vi "Main RLC.vi"() -> ()   [LabVIEW 2017]
uses:
  Types/Parameters Values Type.ctl
  Data Share Type.ctl
  <vilib>/picture/picture.llb/imagedata.ctl
  Types/Parameters Names Type.ctl
  Types/Circuit Type Enum.ctl
  Types/Attachments Type.ctl
  Types/Id Type.ctl
panel:
  out "PUT Response body":string
  out "PUT Responce headers":string
  out "API PUT Endpoint Url Real":string
  out "PUT JSON Payload":string
  in  "API PUT Endpoint Url Pattern":string="https://api.dev.enlil.io/api/v1/document_revisions/external/document-revision-id"
  out "Serial file POST Responce headers":string
  out "Parallel file POST Responce headers":string
  in  "API POST Endpoint Url":string="https://api.dev.enlil.io/api/v1/attachments/external/upload"
  in  "Post Button":bool
  in  "Serial circuit fIlepath":path=path "E:/upwork/Labview-REST-API/serial.png"
  in  "Parallel circuit fIlepath":path=path "E:/upwork/Labview-REST-API/parallel.png"
  in  "Save Button":bool
  out "Serial - Frequency Response Picture":picture
  out "Parallel - Frequency Response Picture":picture
  in  "Calculate Button":bool
  out "Parameters Values":T1
  in  "API Token":string="apitoken 2096a662-4947-42f5-97bc-84cfdf20fe4e:bc240510-8f48-43e3-889a-471659905c2e"
  in  "API GET Endpoint Url":string="https://api.dev.enlil.io/api/v1/document_revisions/external/ALI00017/draft"
  in  "Get Button":bool
  in  "Close Button":bool
  # "1. GET request to receive filter parameters"
  # "2. Calculate Parallel/Serial circuits frequency responce"
  # "3. Save to file"
  # "4. POST/PUT requests to send images"
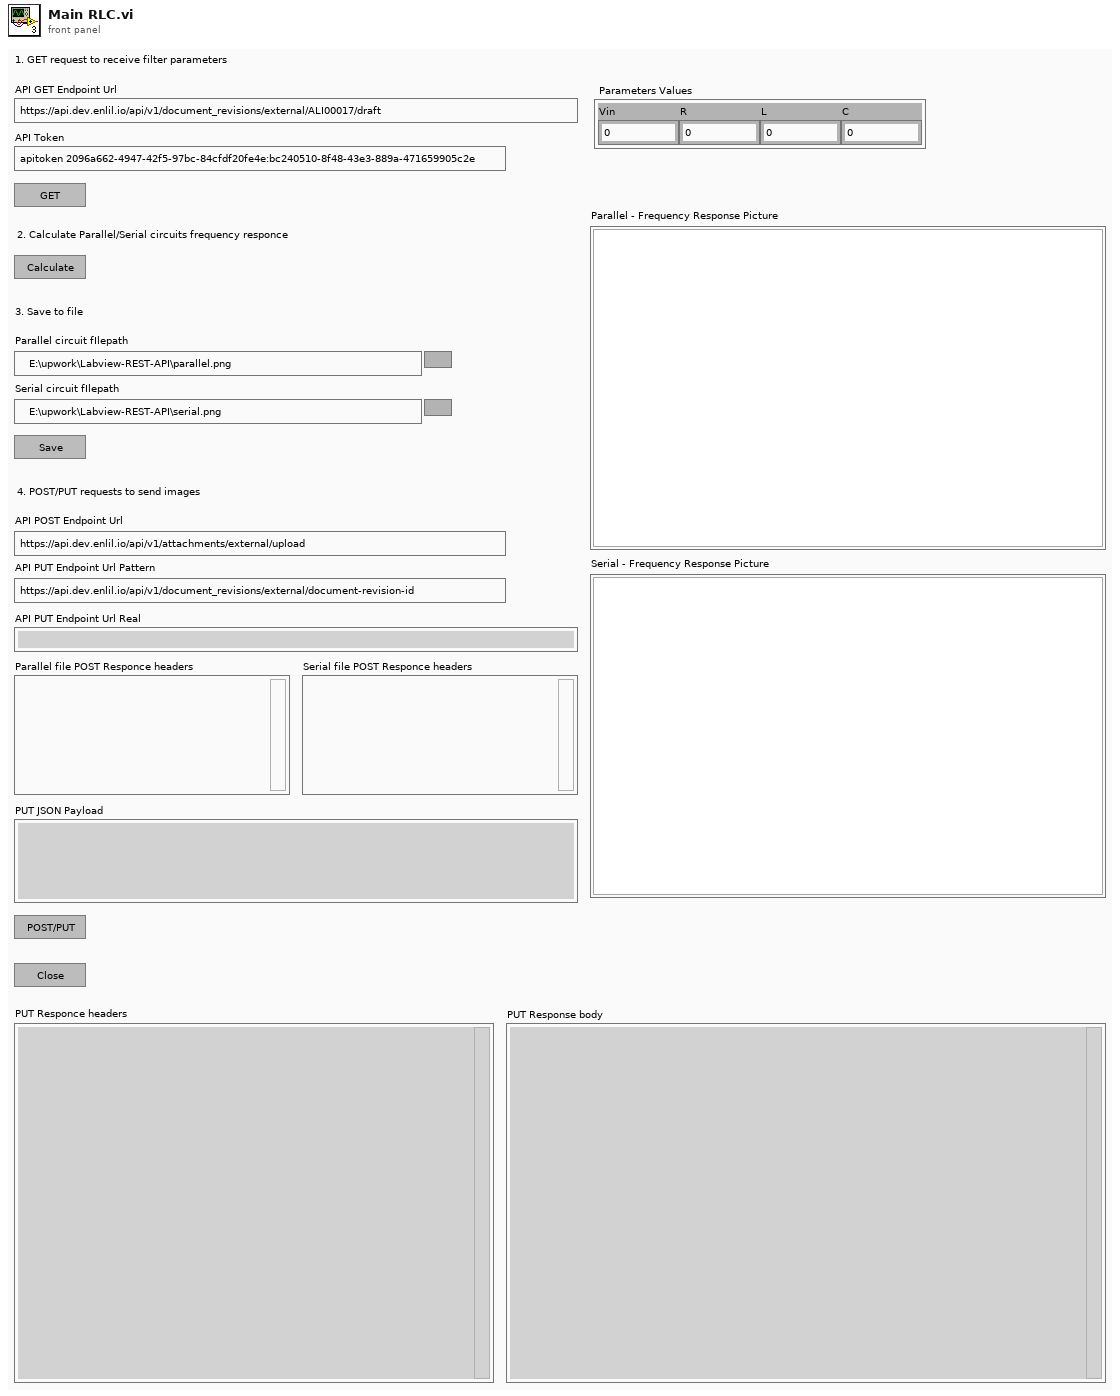
[diagram p1: front panel]
types:
  T1 = typedef "Parameters Values Type.ctl" = cluster{"Vin":dbl, "R":dbl, "L":dbl, "C":dbl}
  T2 = typedef "Data Share Type.ctl" = cluster{"Parallel Image Data":T3, "Serial Image Data":T3, "Parameters Values":T1, "Parallel circuit fIlepath":path, "Serial circuit fIlepath":path, "Document Id":string, "Parallel File Id":string, "Serial File Id":string, "Api Token":string}
  T3 = typedef "imagedata.ctl" = cluster{"image type":i32, "image depth":i32, "image":u8[], "mask":u8[], "colors":u32[], "Rectangle":cluster{"left":i16, "top":i16, "right":i16, "bottom":i16}}
  T4 = typedef "Parameters Names Type.ctl" = cluster{"Vin":string, "R":string, "L":string, "C":string}
  T5 = typedef "Circuit Type Enum.ctl" = enum16{"Parallel", "Serial"}
  T6 = typedef "Id Type.ctl" = cluster{"id":string}
  T7 = typedef "Attachments Type.ctl" = cluster{"attachments":T6[]}
  T8 = typedef "Body Parameter Type.ctl" = cluster{"Name":string, "Value":string}
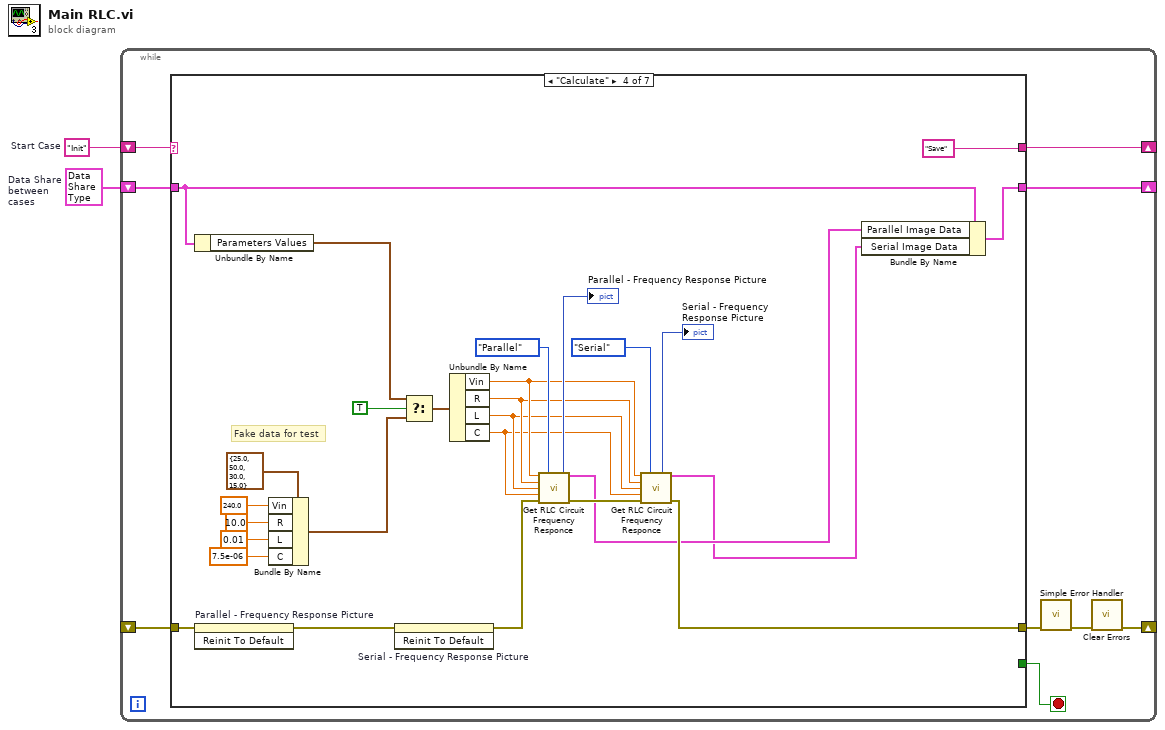
[diagram p0: block diagram]
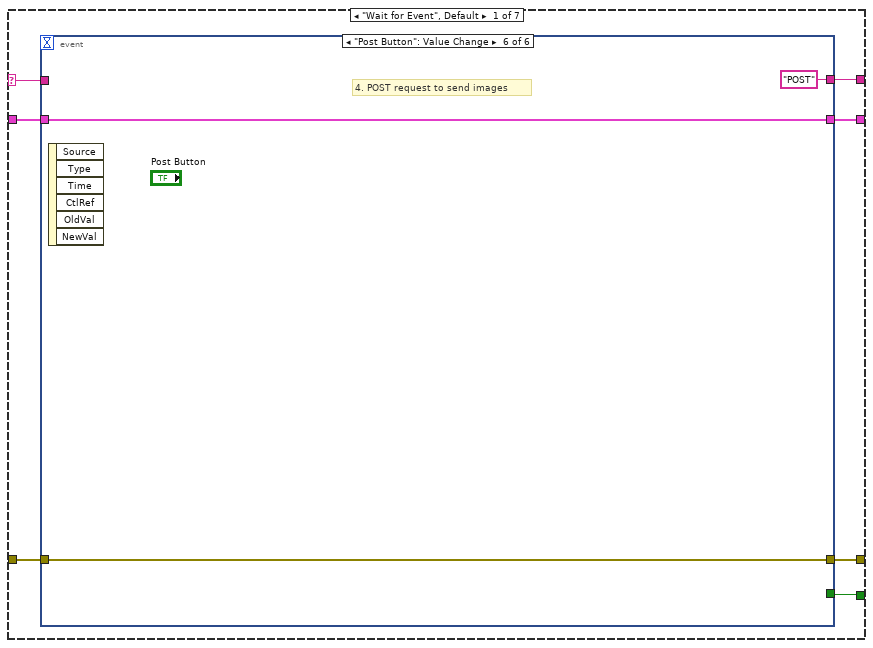
[diagram p2: hidden frame]
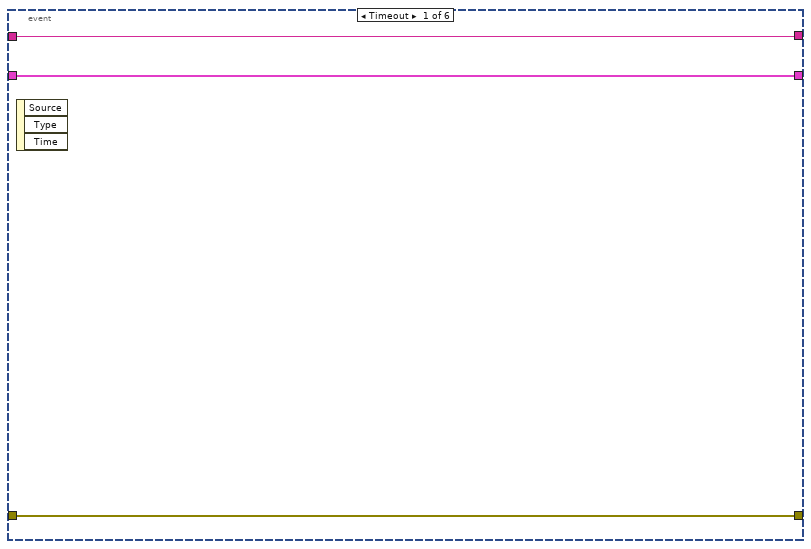
[diagram p3: hidden frame]
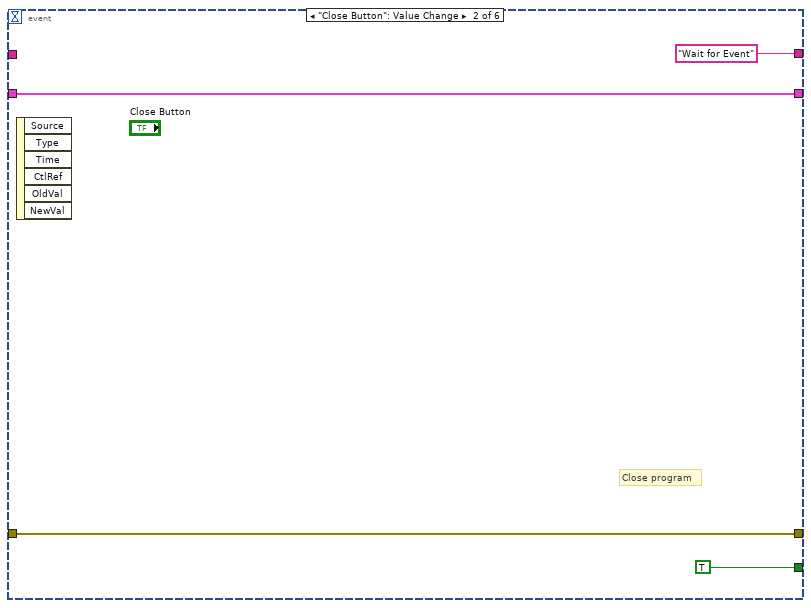
[diagram p4: hidden frame]
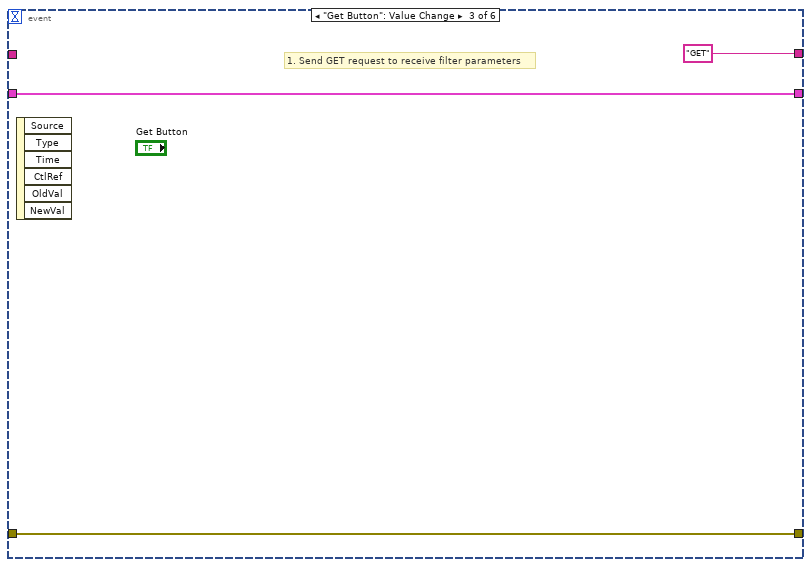
[diagram p5: hidden frame]
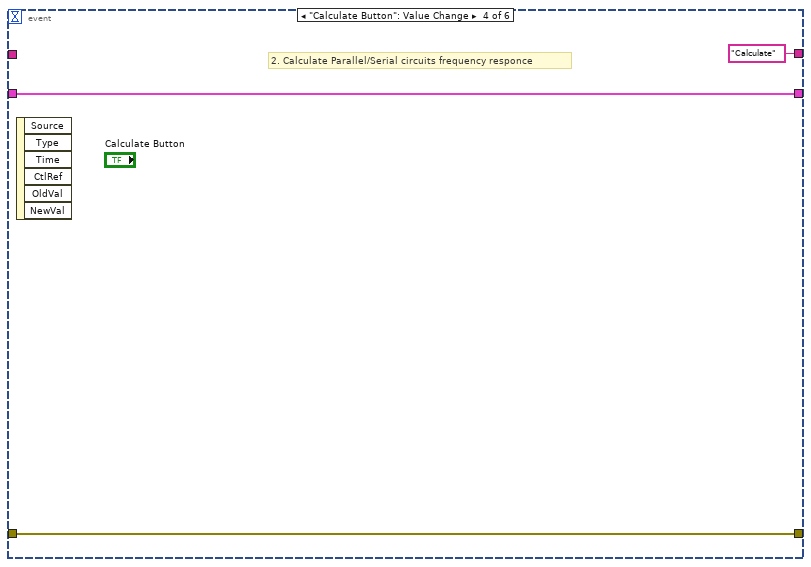
[diagram p6: hidden frame]
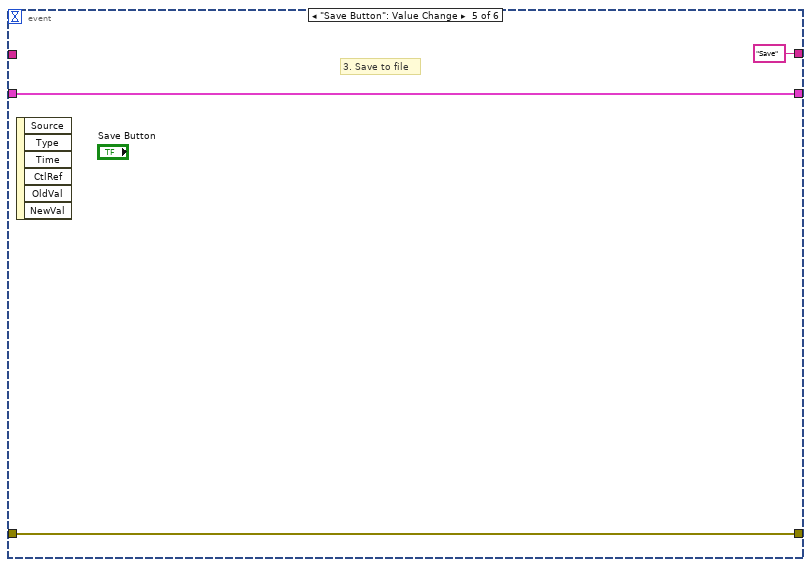
[diagram p7: hidden frame]
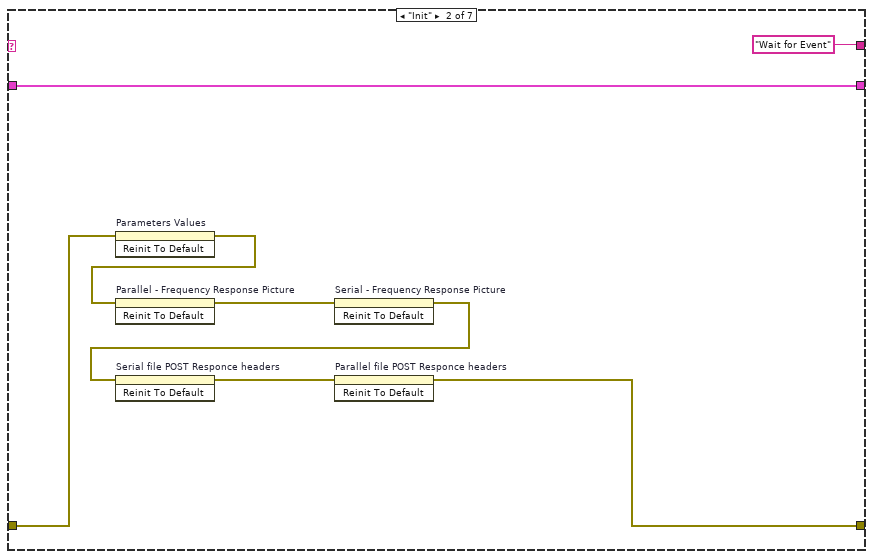
[diagram p8: hidden frame]
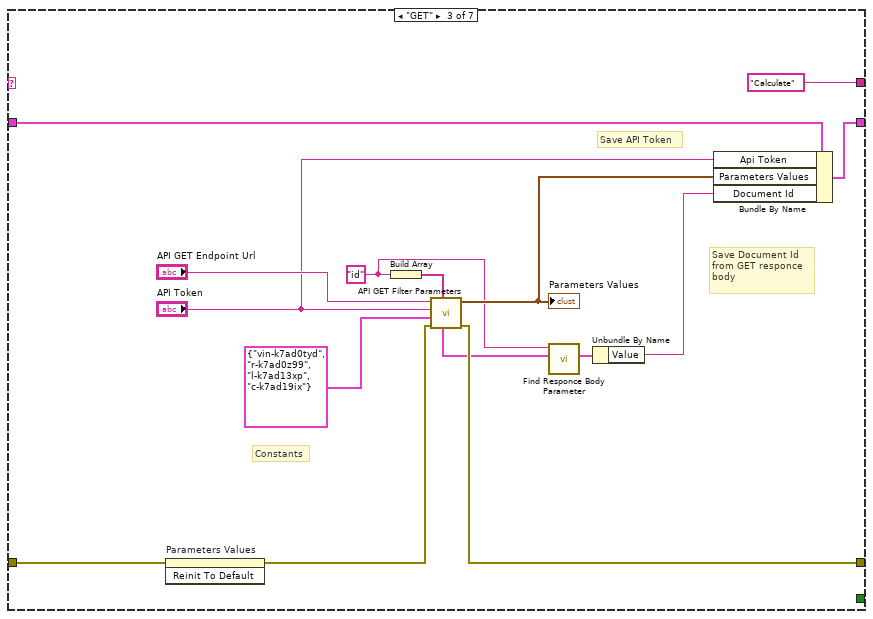
[diagram p9: hidden frame]
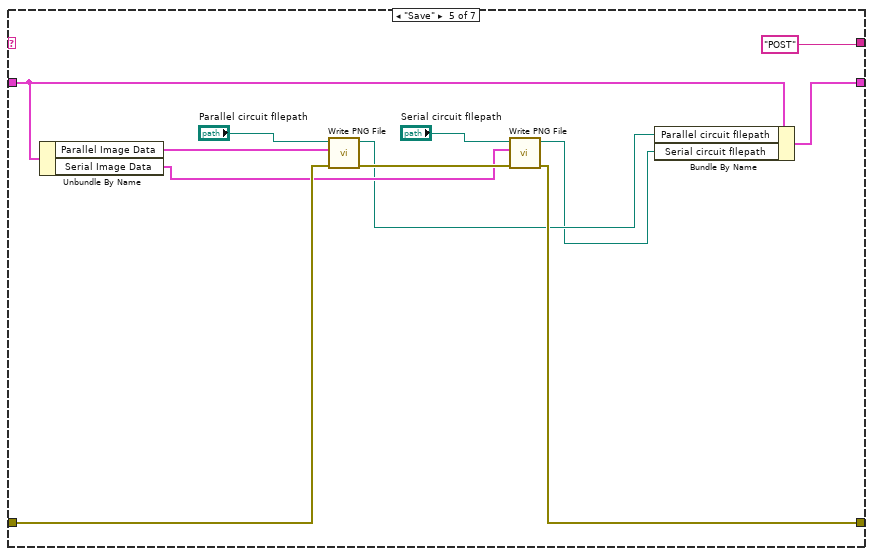
[diagram p10: hidden frame]
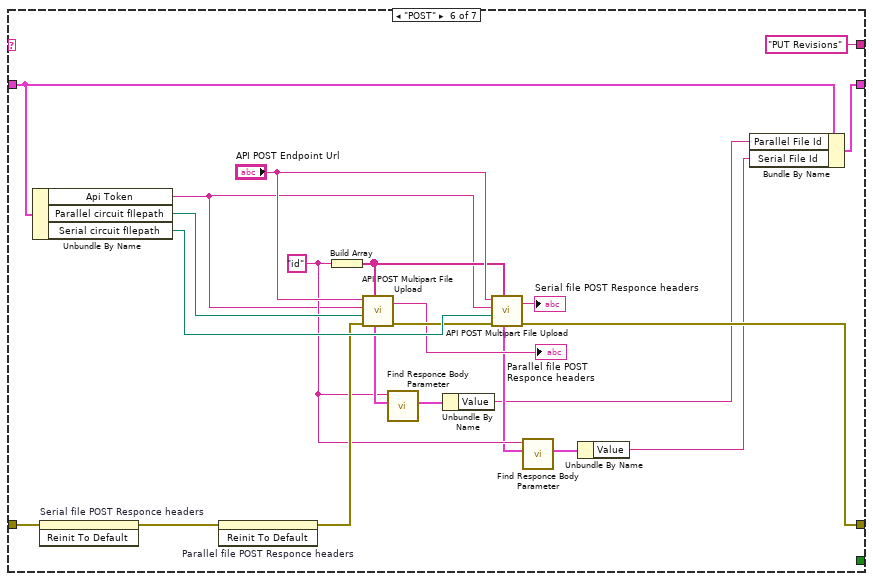
[diagram p11: hidden frame]
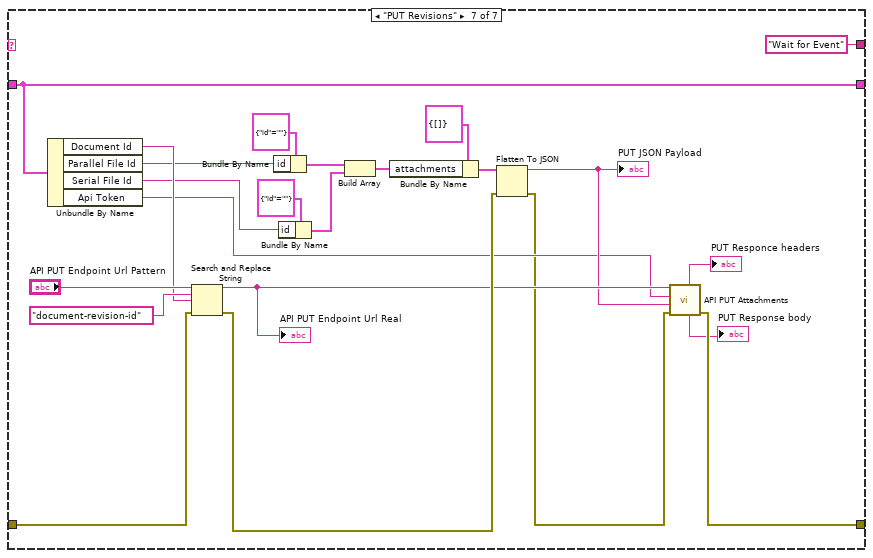
[diagram p12: hidden frame]
diagram:
  w1 = T2 {"Parallel Image Data"={"image type"=0, "image depth"=0, "image"=[], "mask"=[], "colors"=[], "Rectangle"={"left"=0, "top"=0, "right"=0, "bottom"=0}}, "Serial Image Data"={"image type"=0, "image depth"=0, "image"=[], "mask"=[], "colors"=[], "Rectangle"={"left"=0, "top"=0, "right"=0, "bottom"=0}}, "Parameters Values"={"Vin"=0.0, "R"=0.0, "L"=0.0, "C"=0.0}, "Parallel circuit fIlepath"=path "D:/upwork/Labview-REST-API/parallel.png", "Serial circuit fIlepath"=path "D:/upwork/Labview-REST-API/serial.png", "Document Id"="", "Parallel File Id"="", "Serial File Id"="", "Api Token"=""}  # Data Share between  cases
  w2 = "Init"  # Start Case
  n1 = while {
    shift-right: [w9] -> _
    shift-left: w2 -> [w11]
    shift-right: [w5] -> _
    shift-left: _ -> [w8]
    shift-right: [w3] -> _
    shift-left: w1 -> [w4]
    stop <- w10 stop-if-true
    n2 = case shown="\"Calculate\"" w11 {
      selector: w11 -> [w17 _ _ _ _ _ _]
      tunnel: [w18 _ _ _ _ _ _] -> w10
      tunnel: [w16 "Wait for Event" "Calculate" "Save" "POST" "PUT Revisions" "Wait for Event"] -> w9
      tunnel: [w14 w38 w57 w83 w92 w116 w124] -> w7
      tunnel: w8 -> [w15 w44 w56 w82 w96 w113 w130]
      tunnel: w4 -> [w13 w42 w54 w64 w90 w104 w141]
      tunnel: [w12 w42 w53 w63 w91 w103 w141] -> w3
      frame "Wait for Event", Default {
        n3 = event shown="[5] \"Post Button\": Value Change" {
          selector: _ -> [_ _ _ _ _ _]
          dyn-events: _ -> [_ _ _ _ _ _]
          timeout: _ -> [_ _ _ _ _ _]
          tunnel: [_ TRUE _ _ _ _] -> w18
          tunnel: w17 -> [w21 _ _ _ _ _]
          tunnel: [w21 "Wait for Event" "GET" "Calculate" "Save" "POST"] -> w16
          tunnel: w15 -> [w20 w23 w27 w30 w32 w35]
          tunnel: [w20 w23 w27 w30 w32 w35] -> w14
          tunnel: w13 -> [w19 w22 w26 w29 w33 w36]
          tunnel: [w19 w22 w26 w29 w33 w36] -> w12
          event Timeout {
            n4 = event-data() -> ()  [unwired: 1 in, 3 out]
          }
          event "Close Button": Value Change {
            # "Close program"
            n5 = event-data() -> ()  [unwired: 1 in, 6 out]
          }
          event "Get Button": Value Change {
            # "1. Send GET request to receive filter parameters"
            n6 = event-data() -> ()  [unwired: 1 in, 6 out]
          }
          event "Calculate Button": Value Change {
            # "2. Calculate Parallel/Serial circuits frequency responce"
            n7 = event-data() -> ()  [unwired: 1 in, 6 out]
          }
          event "Save Button": Value Change {
            # "3. Save to file"
            n8 = event-data() -> ()  [unwired: 1 in, 6 out]
          }
          event "Post Button": Value Change {
            # "4. POST request to send images"
            n9 = event-data() -> ()  [unwired: 1 in, 6 out]
          }
        }
      }
      frame "Init" {
        n10 = invoke on="Parameters Values" class="Clust (strict)" method="Reinit To Default"(error in=w44) -> (error out=w41:errorcluster)  [unwired: 2 in, 2 out]
        n11 = invoke on="Parallel - Frequency Response Picture" class="Pict" method="Reinit To Default"(error in=w41) -> (error out=w43:errorcluster)  [unwired: 2 in, 2 out]
        n12 = invoke on="Serial - Frequency Response Picture" class="Pict" method="Reinit To Default"(error in=w43) -> (error out=w39:errorcluster)  [unwired: 2 in, 2 out]
        n13 = invoke on="Serial file POST Responce headers" class="Str" method="Reinit To Default"(error in=w39) -> (error out=w40:errorcluster)  [unwired: 2 in, 2 out]
        n14 = invoke on="Parallel file POST Responce headers" class="Str" method="Reinit To Default"(error in=w40) -> (error out=w38:errorcluster)  [unwired: 2 in, 2 out]
      }
      frame "GET" {
        w49 = "id" ("String")
        # "Save Document Id\nfrom GET responce\nbody"
        # "Save API Token"
        # "Constants"
        n15 = invoke on="Parameters Values" class="Clust (strict)" method="Reinit To Default"(error in=w56) -> (error out=w55:errorcluster)  [unwired: 2 in, 2 out]
        n16 = Build Array(w49) -> (w50:string[])
        n17 = call "API GET Filter Parameters.vi"("Body Parameters Names"=w50, "error in (no error)"=w55, "Filter Parameters Names"=T4 {"Vin"="vin-k7ad0tyd", "R"="r-k7ad0z99", "L"="l-k7ad13xp", "C"="c-k7ad19ix"} ("Parameters Names"), "API Token"="API Token", "API Endpoint Url"="API GET Endpoint Url") -> ("error out"=w57:errorcluster, "Parameters Values"=w52:T1, "Body Parameters out"=w51:T8[])  [unwired: 2 in, 2 out]
        "Parameters Values" <- w52
        n18 = call "Find Responce Body Parameter.vi"("Body Parameters in"=w51, "Parameter name"=w49) -> ("Body Parameter"=w48:T8)  [unwired: 8 in, 1 out]
        n19 = Unbundle By Name(w48) -> ("Value"=w47:string)
        n20 = Bundle By Name(cluster=w54, "Api Token"="API Token", "Parameters Values"=w52, "Document Id"=w47) -> (w53:T2)
      }
      frame "Calculate" {
        # "Fake data for test"
        n21 = Unbundle By Name(w64) -> ("Parameters Values"=w65:T1)
        n22 = invoke on="Parallel - Frequency Response Picture" class="Pict" method="Reinit To Default"(error in=w82) -> (error out=w81:errorcluster)  [unwired: 2 in, 2 out]
        n23 = Bundle By Name(cluster=T1 {"Vin"=25.0, "R"=50.0, "L"=30.0, "C"=15.0} ("Parameters Values"), "Vin"=240.0, "R"=10.0, "L"=0.01, "C"=7.5e-06) -> (w68:T1)
        n24 = invoke on="Serial - Frequency Response Picture" class="Pict" method="Reinit To Default"(error in=w81) -> (error out=w80:errorcluster)  [unwired: 2 in, 2 out]
        n25 = Select(t=w65, s=TRUE, f=w68) -> (s? t:f=w67:T1)
        n26 = Unbundle By Name(w67) -> ("Vin"=w79:dbl, "R"=w78:dbl, "L"=w77:dbl, "C"=w76:dbl)
        n27 = call "Get RLC Circuit Frequency Responce.vi"("Vin amplitude"=w79, "Circuit Type Enum"=Circuit_Type_Enum."Parallel", "Resistence (R)"=w78, "Impedence (H)"=w77, "Capacitave (F)"=w76, "error in (no error)"=w80) -> ("Frequency Response Picture"=→"Parallel - Frequency Response Picture":picture, "Frequency Response Image Data"=w62:T3, "error out"=w84:errorcluster)  [unwired: 6 in, 1 out]
        n28 = call "Get RLC Circuit Frequency Responce.vi"("Vin amplitude"=w79, "Circuit Type Enum"=Circuit_Type_Enum."Serial", "Resistence (R)"=w78, "Impedence (H)"=w77, "Capacitave (F)"=w76, "error in (no error)"=w84) -> ("Frequency Response Picture"=→"Serial - Frequency Response Picture":picture, "Frequency Response Image Data"=w61:T3, "error out"=w83:errorcluster)  [unwired: 6 in, 1 out]
        n29 = Bundle By Name(cluster=w64, "Parallel Image Data"=w62, "Serial Image Data"=w61) -> (w63:T2)
      }
      frame "Save" {
        n30 = Unbundle By Name(w90) -> ("Parallel Image Data"=w97:T3, "Serial Image Data"=w93:T3)
        n31 = call <vilib>:"Write PNG File.vi"("error in (no error)"=w96, "image data"=w97, "path to PNG file"="Parallel circuit fIlepath") -> ("error out"=w95:errorcluster, "path"=w89:path)  [unwired: 7 in]
        n32 = call <vilib>:"Write PNG File.vi"("error in (no error)"=w95, "image data"=w93, "path to PNG file"="Serial circuit fIlepath") -> ("error out"=w92:errorcluster, "path"=w88:path)  [unwired: 7 in]
        n33 = Bundle By Name(cluster=w90, "Parallel circuit fIlepath"=w89, "Serial circuit fIlepath"=w88) -> (w91:T2)
      }
      frame "POST" {
        w106 = "id" ("String")
        n34 = Unbundle By Name(w104) -> ("Api Token"=w100:string, "Parallel circuit fIlepath"=w120:path, "Serial circuit fIlepath"=w118:path)
        n35 = invoke on="Serial file POST Responce headers" class="Str" method="Reinit To Default"(error in=w113) -> (error out=w112:errorcluster)  [unwired: 2 in, 2 out]
        n36 = invoke on="Parallel file POST Responce headers" class="Str" method="Reinit To Default"(error in=w112) -> (error out=w111:errorcluster)  [unwired: 2 in, 2 out]
        n37 = Build Array(w106) -> (w110:string[])
        n38 = call "API POST Multipart File Upload.vi"("Body Parameters Names"=w110, "error in (no error)"=w111, "FIlepath"=w120, "API Token"=w100, "API Endpoint Url"="API POST Endpoint Url") -> ("error out"=w117:errorcluster, "Responce headers"=→"Parallel file POST Responce headers":string, "Body Parameters out"=w109:T8[])  [unwired: 3 in, 1 out]
        n39 = call "Find Responce Body Parameter.vi"("Body Parameters in"=w109, "Parameter name"=w106) -> ("Body Parameter"=w108:T8)  [unwired: 8 in, 1 out]
        n40 = Unbundle By Name(w108) -> ("Value"=w102:string)
        n41 = call "API POST Multipart File Upload.vi"("Body Parameters Names"=w110, "error in (no error)"=w117, "FIlepath"=w118, "API Token"=w100, "API Endpoint Url"="API POST Endpoint Url") -> ("error out"=w116:errorcluster, "Responce headers"=→"Serial file POST Responce headers":string, "Body Parameters out"=w105:T8[])  [unwired: 3 in, 1 out]
        n42 = call "Find Responce Body Parameter.vi"("Body Parameters in"=w105, "Parameter name"=w106) -> ("Body Parameter"=w107:T8)  [unwired: 8 in, 1 out]
        n43 = Unbundle By Name(w107) -> ("Value"=w101:string)
        n44 = Bundle By Name(cluster=w104, "Parallel File Id"=w102, "Serial File Id"=w101) -> (w103:T2)
      }
      frame "PUT Revisions" {
        n45 = Unbundle By Name(w141) -> ("Document Id"=w140:string, "Parallel File Id"=w137:string, "Serial File Id"=w135:string, "Api Token"=w126:string)
        n46 = Search and Replace String(input string="API PUT Endpoint Url Pattern", search string="document-revision-id", replace string=w140, error in=w130) -> (result string=w128:string, error out=w129:errorcluster)  [unwired: 4 in, 2 out]
        "API PUT Endpoint Url Real" <- w128
        n47 = Bundle By Name(cluster=T6 {"id"=""} ("Id Type"), "id"=w137) -> (w134:T6)
        n48 = Bundle By Name(cluster=T6 {"id"=""} ("Id Type"), "id"=w135) -> (w133:T6)
        n49 = Build Array(w134, w133) -> (w132:T6[])
        n50 = Bundle By Name(cluster=T7 {"attachments"=[]} ("Attachments Type"), "attachments"=w132) -> (w131:T7)
        n51 = Flatten To JSON(anything=w131, error in (no error)=w129) -> (JSON string=w127:string, 11:w125:errorcluster)  [unwired: 1 in]
        "PUT JSON Payload" <- w127
        n52 = call "API PUT Attachments.vi"("error in (no error)"=w125, "Buffer"=w127, "API Token"=w126, "API Endpoint Url"=w128) -> ("error out"=w124:errorcluster, "Response body"=→"PUT Response body":string, "Responce headers"=→"PUT Responce headers":string)  [unwired: 5 in]
      }
    }
    n53 = call <vilib>:"Simple Error Handler.vi"("error in (no error)"=w7) -> ("error out"=w6:errorcluster)  [unwired: 4 in, 4 out]
    n54 = call <vilib>:"Clear Errors.vi"("error in (no error)"=w6) -> ("error out"=w5:errorcluster)  [unwired: 5 in, 1 out]
  }
